vi "backwards.vi"(7 "Parâmetros Ini 2":T2={"Gyro Port"=0, "Sensor - Left"=3, "Sensor - Right"=2, "     Color \nSensor Port"=1, "Kp Front"=0.5, "Motor speed"=-15, "Distance to street"=0.0, "Motor speed turns"=16, "Kp Curvas"=0.0} {"Kp Front" format="%.3f"; "Color \nSensor Port" items=["Port 1", "Port 2", "Port 3", "Port 4"]; "Sensor - Right" items=["Port 1", "Port 2", "Port 3", "Port 4"]; "Sensor - Left" items=["Port 1", "Port 2", "Port 3", "Port 4"]; "Gyro Port" items=["Port 1", "Port 2", "Port 3", "Port 4"]}, 8 "NXT/EV3":T1, 10 "Características Ini":T5={"Colors and Directions"=[enum."Zero", enum."Zero", enum."Zero", enum."Zero", enum."Zero", enum."Zero"], "Direction"=enum."Right", "CS"=enum."Street", "Old Color"=enum."White"}, 11 "First Angle":sgl) -> (1 "NXT/EV3 2":T1)   [LabVIEW 2016]
uses:
  <vilib>/NXT/Subs/LVHSConnector.ctl
  <vilib>/NXT/LegoClasses/BrickReference/BrickReference.lvclass
  <vilib>/NXT/Subs/ColorSensorColors.ctl
  parametros.ctl
  <vilib>/NXT/Block Support/NXT_InputPort.ctl
  <vilib>/NXT/Block Support/NXT_OutputPort.ctl
  <vilib>/NXT/Dual Mode Library/Sensors/EV3_Gyro_Angle.vi
  <vilib>/NXT/NXTIO Xnodes/NXTIONodeSubVIs/NXTMoveMotors.vi
  <vilib>/NXT/NXTIO Xnodes/AddressXNode/NXTIOAddress.xnode
  <vilib>/NXT/NXTIO Xnodes/NXTIOXNode/NXTIO.xnode
panel:
  out "Degrees 2":sgl
  # "black"
  # "blue"
  # "green"
  # "yellow"
  # "red"
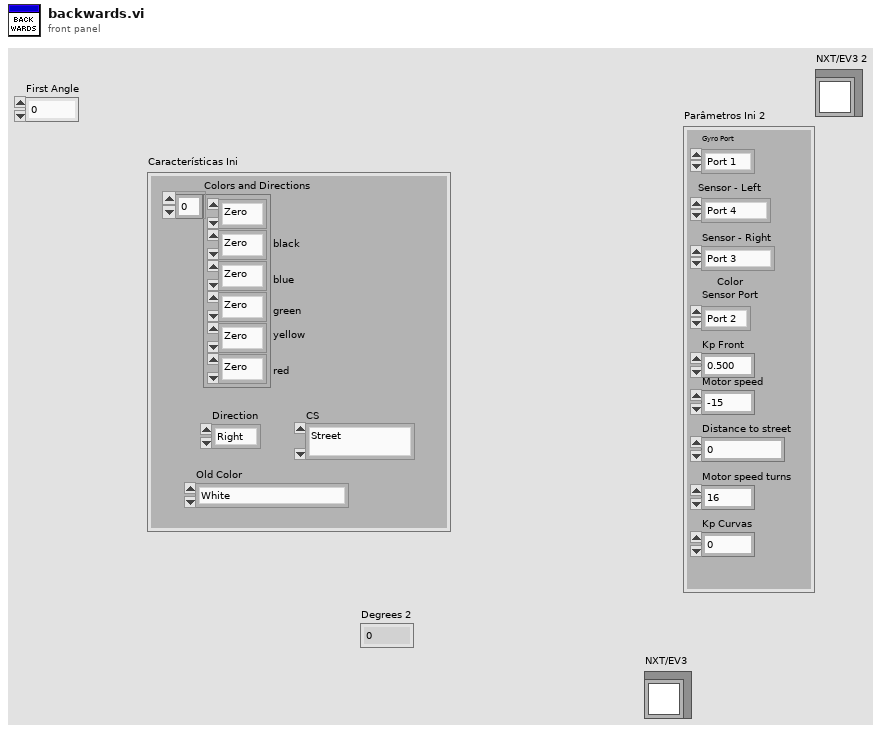
[diagram p1: front panel]
types:
  T1 = typedef "LVHSConnector.ctl" = refnum<class "BrickReference.lvclass">
  T2 = typedef "parametros.ctl" = cluster{"Gyro Port":T3, "Sensor - Left":T3, "Sensor - Right":T3, "     Color \nSensor Port":T3, "Kp Front":dbl, "Motor speed":i32, "Distance to street":dbl, "Motor speed turns":i32, "Kp Curvas":dbl}
  T3 = typedef "NXT_InputPort.ctl" = u32
  T4 = typedef "ColorSensorColors.ctl" = enum16{"No Color", "Black", "Blue", "Green", "Yellow", "Red", "White", "Brown"}
  T5 = cluster{"Colors and Directions":enum16{"Zero", "Right", "Front", "Left"}[], "Direction":enum16{"Zero", "Right", "Front", "Left"}, "CS":enum16{"Street", "Intersection", "End", "Stop", "Square", "Delivery"}, "Old Color":T4}
  T6 = typedef "NXT_OutputPort.ctl" = u8
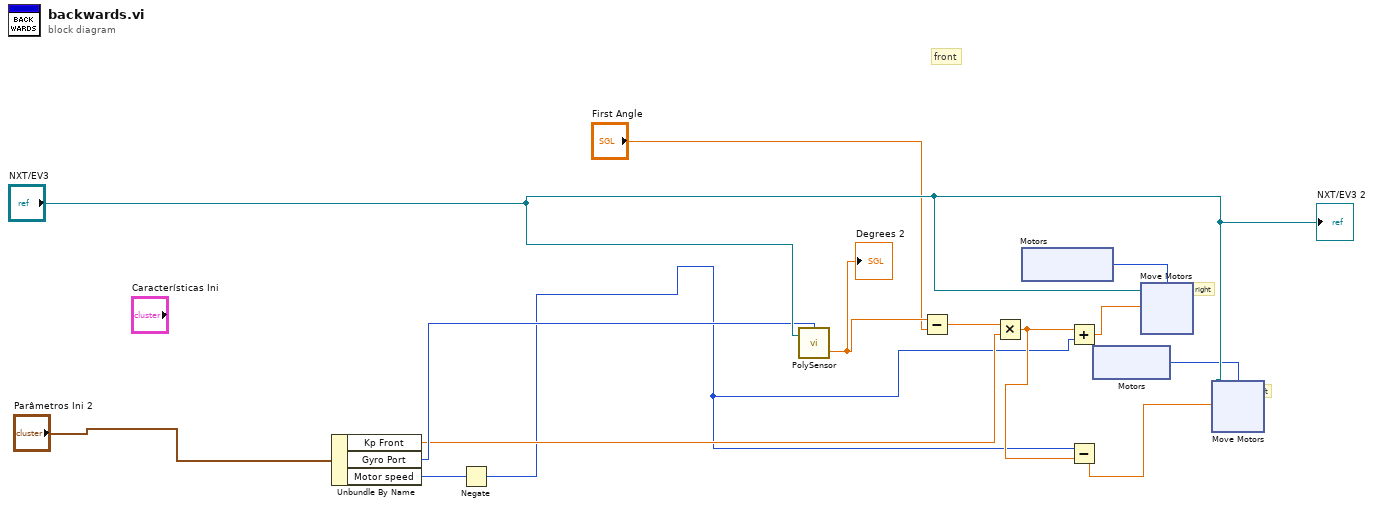
[diagram p0: block diagram]
diagram:
  # "left"
  # "right"
  # "front"
  n1 = Unbundle By Name("Parâmetros Ini 2") -> ("Kp Front"=w4:dbl, "Gyro Port"=w13:T3, "Motor speed"=w2:i32)
  n2 = Negate(x=w2) -> (-x=w1:i32)
  n3 = call-poly <vilib>:"PolySensor.vi"("NXT/EV3"="NXT/EV3", "Port (Port 1)"=w13) -> ("Degrees"=w9:sgl)  [unwired: 1 in, 1 out]
  "Degrees 2" <- w9
  n4 = Subtract(x=w9, y="First Angle") -> (x-y=w10:sgl)
  n5 = Multiply(x=w10, y=w4) -> (x*y=w11:dbl)
  n6 = xnode "Motors"() -> ("Motor"=w7:T6)
  n7 = Add(x=w11, y=w1) -> (x+y=w12:dbl)
  n8 = Subtract(x=w1, y=w11) -> (x-y=w8:dbl)
  n9 = xnode "Motors"() -> ("Motor"=w6:T6)
  n10 = xnode "Move Motors"("Power/Speed 1"=w12, "Motors"=w7, "NXT/EV3"="NXT/EV3") -> ()  [unwired: 1 out]
  n11 = xnode "Move Motors"("Power/Speed 1"=w8, "Motors"=w6, "NXT/EV3"="NXT/EV3") -> ()  [unwired: 1 out]
  "NXT/EV3 2" <- "NXT/EV3"
